vi "Get SLSC Module By Slot.vi"(8 "error in (no error)":errorcluster, 10 "Slot":u32=1, 11 "SLSC Chassis":u64) -> (0 "error out":errorcluster, 2 "SLSC Module":u64, 3 "SLSC Chassis out":u64)   [LabVIEW 2020, in "VeriStand SLSC Scripting.lvlib"]
uses:
  VeriStand SLSC Scripting.lvlib
  NationalInstruments.VeriStand.SystemDefinitionAPI
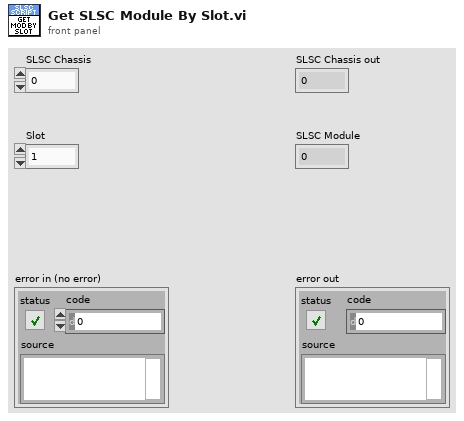
[diagram p1: front panel]
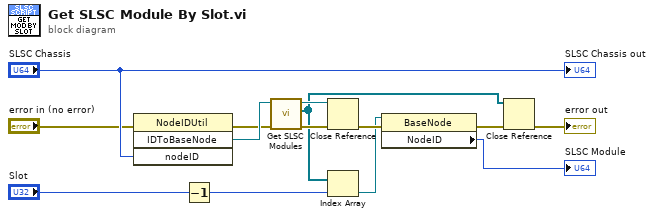
[diagram p0: block diagram]
diagram:
  n1 = invoke class="NodeIDUtil" method="IDToBaseNode"(error in="error in (no error)", "nodeID"="SLSC Chassis") -> (error out=w1:errorcluster, "IDToBaseNode"=w14:refnum<k24>)  [unwired: 2 in, 2 out]
  n2 = Decrement(x="Slot") -> (x-1=w7:u32)
  n3 = call "Get SLSC Modules.vi"("error in (no error)"=w1, "SLSC Chassis"=w14) -> ("error out"=w11:errorcluster, "SLSC Modules"=w3:refnum<k24>[], "SLSC Chassis out"=w9:refnum<k24>)  [unwired: 7 in]
  n4 = Close Reference(reference=w9, error in (no error)=w11) -> (error out=w10:errorcluster)
  n5 = Index Array(array=w3, index=w7) -> (element=w6:refnum<k24>)
  n6 = property class="BaseNode"(reference=w6, error in=w10) -> (error out=w5:errorcluster, "NodeID"=→"SLSC Module":u64)  [unwired: 1 out]
  n7 = Close Reference(reference=w3, error in (no error)=w5) -> (error out=→"error out":errorcluster)
  "SLSC Chassis out" <- "SLSC Chassis"
